vi "Set Target.vi"(8 "error in (no error)":errorcluster, 9 "Target Rate (T/min)":dbl, 10 "Target Field (T)":dbl, 11 "Instrument.Oxford1820 in":refnum<class "Instrument.Oxford1820.lvclass">) -> (0 "error out":errorcluster, 3 "Instrument.Oxford1820 out":refnum<class "Instrument.Oxford1820.lvclass">)   [LabVIEW 2016, in "Instrument.Oxford1820.lvclass"]
uses:
  Instrument.Oxford1820.lvclass
  Typedefs/Targets.ctl
  Typedefs/Instrument.Oxford1820.Commands-enum.ctl
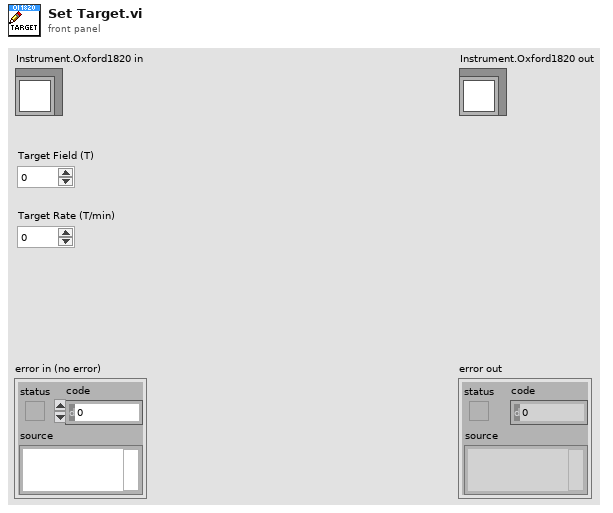
[diagram p1: front panel]
types:
  T1 = typedef "Instrument.Oxford1820.lvclass/Instrument.Oxford1820.Commands-enum.ctl" = enum16{"setAction", "setTarget", "setSwitchHeat", "setLambda", "setFillMode", "setNeedleValve", "setMagnetField", "getStatus", "getTarget", "getSwitchHeat", "getPSUField", "getMagnetField"}
  T2 = typedef "Instrument.Oxford1820.lvclass/Targets.ctl" = cluster{"Field (T)":dbl, "Field Rate (T/min)":dbl}
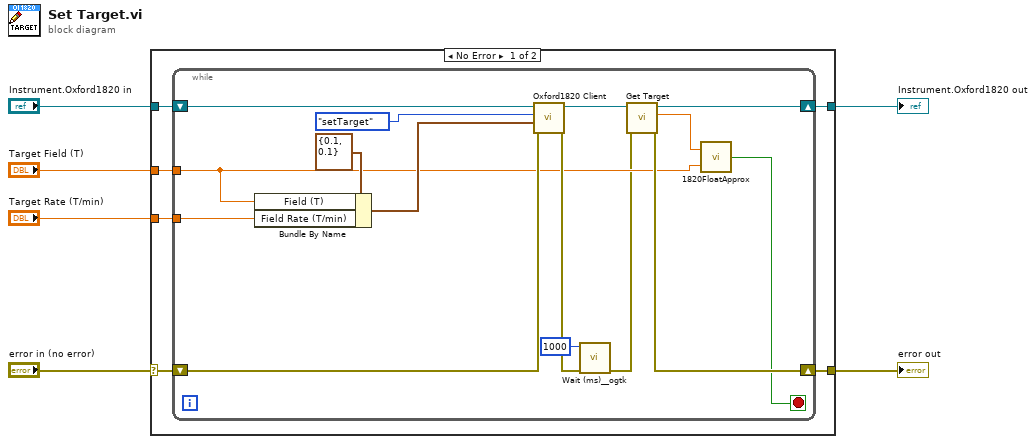
[diagram p0: block diagram]
diagram:
  n1 = case shown="No Error" "error in (no error)" {
    selector: "error in (no error)" -> [w9 w29]
    tunnel: "Target Rate (T/min)" -> [w12 _]
    tunnel: [w7 w29] -> w5
    tunnel: "Target Field (T)" -> [w11 _]
    tunnel: "Instrument.Oxford1820 in" -> [w10 w28]
    tunnel: [w8 w28] -> w1
    frame No Error {
      n2 = while {
        tunnel: w12 -> [w27]
        tunnel: w11 -> [w16]
        shift-right: [w20] -> w8
        shift-left: w10 -> [w25]
        shift-right: [w18] -> w7
        shift-left: w9 -> [w22]
        stop <- w15 stop-if-true
        n3 = Bundle By Name(cluster=T2 {"Field (T)"=0.1, "Field Rate (T/min)"=0.1} ("Mercury Targets"), "Field (T)"=w16, "Field Rate (T/min)"=w27) -> (w23:T2)
        n4 = call "Oxford1820 Client.vi"("error in (no error)"=w22, "Data"=w23, "Commands"=Instrument.Oxford1820.Commands-enum."setTarget", "Instrument.1820 in"=w25) -> ("error out"=w19:errorcluster, "Instrument.1820 out"=w21:refnum<class "Instrument.Oxford1820.lvclass">)  [unwired: 5 in, 1 out]
        n5 = call <userlib>:"Wait (ms)__ogtk.vi"("error in (no error)"=w19, "milliseconds to wait"=u32 1000) -> ("error out"=w14:errorcluster)  [unwired: 8 in, 1 out]
        n6 = call-dynamic "Get Target.vi"("error in (no error)"=w14, "Instrument.Oxford1820 in"=w21) -> ("error out"=w18:errorcluster, "Target Field (T)"=w17:dbl, "Instrument.Oxford1820 out"=w20:refnum<class "Instrument.Oxford1820.lvclass">)  [unwired: 6 in, 1 out]
        n7 = call "1820FloatApprox.vi"("y"=w16, "x"=w17) -> ("x ~ y?"=w15:bool)
      }
    }
    frame Error {
    }
  }
  "Instrument.Oxford1820 out" <- w1
  "error out" <- w5
